vi "ResetFrontPanel.vi"(8 "Error In":errorcluster, 11 "VI Ref In":refnum<vi>) -> (0 "Error Out":errorcluster, 3 "VI Ref Out":refnum<vi>)   [LabVIEW 2012, in "LV-Utilities.lvlib"]
uses:
  LV-Utilities.lvlib
  <vilib>/Utility/miscctls.llb/LVPointTypeDef.ctl
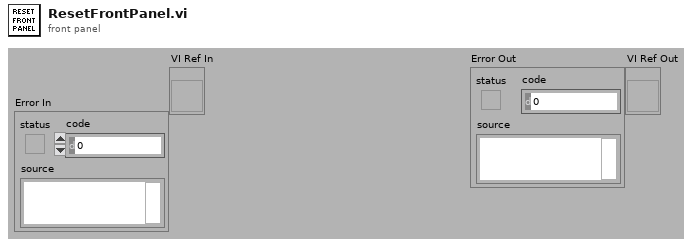
[diagram p1: front panel]
types:
  T1 = typedef "LVPointTypeDef.ctl" = cluster{"Horizontal":i16, "Vertical":i16}
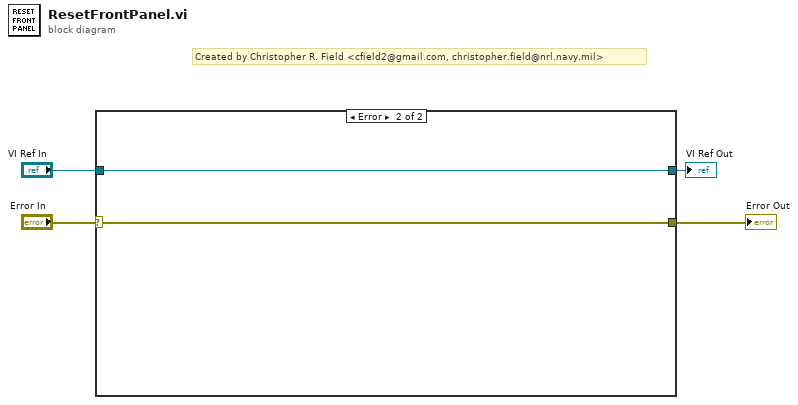
[diagram p0: block diagram]
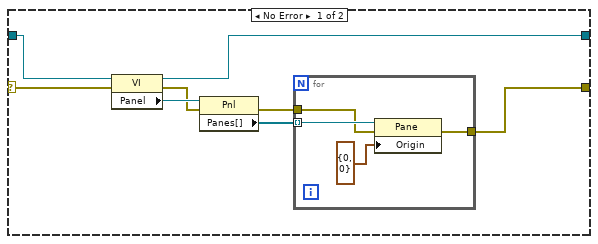
[diagram p2: hidden frame]
diagram:
  # "Created by Christopher R. Field <cfield2@gmail.com, christopher.field@nrl.navy.mil>"
  n1 = case shown="Error" "Error In" {
    selector: "Error In" -> [w7 w18]
    tunnel: [w5 w18] -> w4
    tunnel: "VI Ref In" -> [w8 w17]
    tunnel: [w6 w17] -> w1
    frame No Error {
      n2 = property class="VI"(reference=w8, error in=w7) -> (reference out=w6:refnum<vi>, error out=w11:errorcluster, "Panel"=w12:refnum<vi>)
      n3 = property class="Pnl"(reference=w12, error in=w11) -> (error out=w9:errorcluster, "Panes[]"=w10:refnum<vi>[])  [unwired: 1 out]
      n4 = for {
        tunnel: w10 -> [w16] mode=indexing
        tunnel: w9 -> [w14]
        tunnel: [w13] -> w5
        n5 = property class="Pane"(reference=w16, error in=w14, "Origin"=T1 {"Horizontal"=0, "Vertical"=0}) -> (error out=w13:errorcluster)  [unwired: 1 out]
      }
    }
    frame Error {
    }
  }
  "Error Out" <- w4
  "VI Ref Out" <- w1
